vi "LED Control.vi"(9 "D-Pad":T1, 10 "Axes":T2) -> ()   [LabVIEW 2017]
uses:
  Common Code/Gamepads/Axes Cluster.ctl
  Common Code/Gamepads/D-Pad.ctl
  Robot Global Data.vi
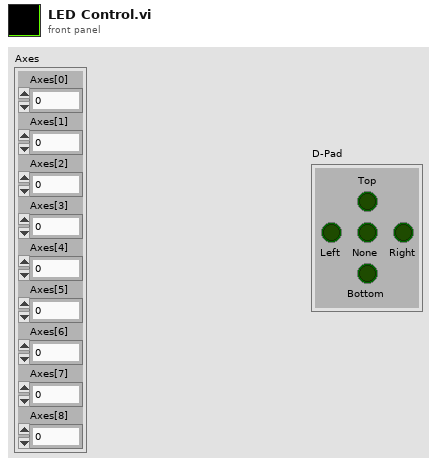
[diagram p1: front panel]
types:
  T1 = typedef "D-Pad.ctl" = cluster{"Top":bool, "Bottom":bool, "None":bool, "Right":bool, "Left":bool}
  T2 = typedef "Axes Cluster.ctl" = cluster{"Axes[0]":dbl, "Axes[1]":dbl, "Axes[2]":dbl, "Axes[3]":dbl, "Axes[4]":dbl, "Axes[5]":dbl, "Axes[6]":dbl, "Axes[7]":dbl, "Axes[8]":dbl}
  T3 = typedef "LED Command Cluster.ctl" = cluster{"DriverRED":bool, "DriverBLUE":bool, "Saboi":bool}
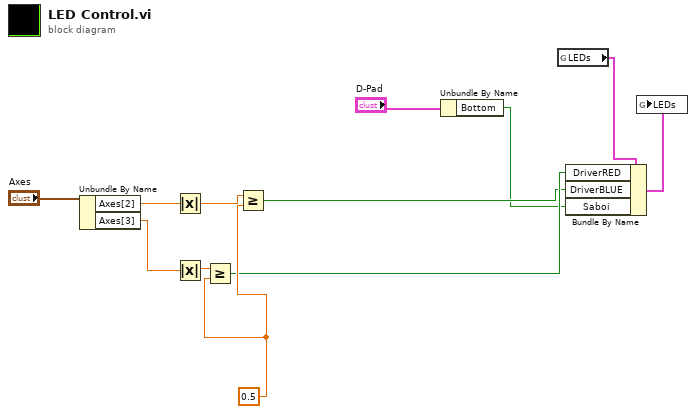
[diagram p0: block diagram]
diagram:
  w4 = 0.5
  n1 = Unbundle By Name("Axes") -> ("Axes[2]"=w8:dbl, "Axes[3]"=w7:dbl)
  n2 = Absolute Value(x=w8) -> (abs(x)=w6:dbl)
  n3 = Absolute Value(x=w7) -> (abs(x)=w5:dbl)
  n4 = Greater Or Equal?(x=w5, y=w4) -> (x >= y?=w3:bool)
  n5 = Greater Or Equal?(x=w6, y=w4) -> (x >= y?=w2:bool)
  n6 = Unbundle By Name("D-Pad") -> ("Bottom"=w1:bool)
  n7 = global read "Robot Global Data.vi" "LEDs"() -> (w10:T3)
  n8 = Bundle By Name(cluster=w10, "DriverRED"=w3, "DriverBLUE"=w2, "Saboi"=w1) -> (w9:T3)
  n9 = global write "Robot Global Data.vi" "LEDs"(w9) -> ()
